vi "DWF MSO Init AtoD.vi"() -> (0 "Error Out":errorcluster, 3 "Instrument Handle Out":u32)   [LabVIEW 2024]
uses:
  <vilib>/DigilentWF/DigilentWF.lvlib
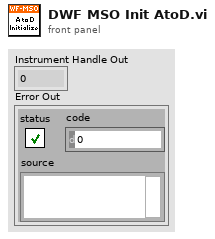
[diagram p1: front panel]
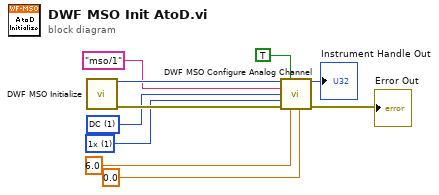
[diagram p0: block diagram]
diagram:
  w7 = 1 items=["AC", "DC"] ("Vertical Coupling")
  w8 = 1 items=["1x"=1, "10x"=10] ("Probe Attenuation")
  n1 = call <vilib>:"DWF MSO Initialize.vi"() -> ("Instrument Handle Out"=w10:u32, "Error Out"=w9:errorcluster)  [unwired: 14 in]
  n2 = call <vilib>:"DWF MSO Configure Analog Channel.vi"("Instrument Handle In"=w10, "Enable Channel"=TRUE, "Channel"="mso/1", "Vertical Coupling"=w7, "Probe Attenuation"=w8, "Error In"=w9, "Vertical Range"=6.0, "Vertical Offset"=0.0) -> ("Instrument Handle Out"=→"Instrument Handle Out":u32, "Error Out"=→"Error Out":errorcluster)  [unwired: 6 in]
